vi "Open Text Log File.vi"(7 "Text Log File Type":refnum<class "Text Log File.lvclass">, 8 "error in (no error)":errorcluster, 9 "Disable Buffering (F)":bool, 10 "Operation":T1, 11 "File Path":path) -> (0 "error out":errorcluster, 3 "Text Log File out":refnum<class "Text Log File.lvclass">)   [LabVIEW 2015, in "Text Log File.lvclass"]
doc: "Opens a text file. Translate the file operation to the expected format and open the file. Set the file position to the end of the file in case we are appending to an existing file."
uses:
  Text Log File.lvclass
  Log File/Operation.ctl
  Log File/Log File Type.ctl
  Log File/Log File.lvclass/Log File.ctl
  Text Log File.lvclass/Text Log File.ctl
  Log File/Log File.lvclass
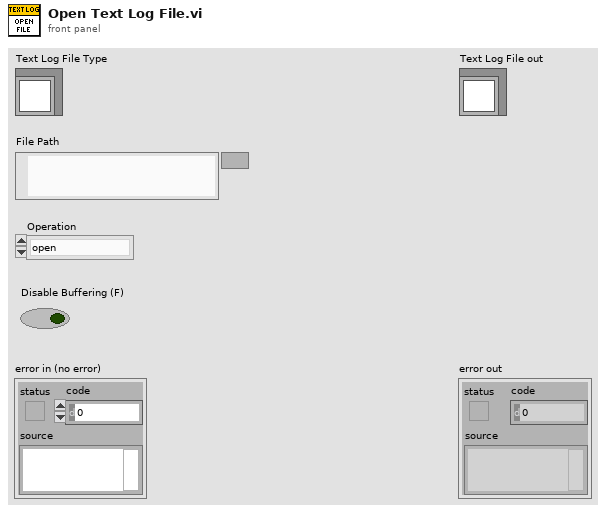
[diagram p1: front panel]
types:
  T1 = typedef "Log File.lvclass/Operation.ctl" = enum16{"open", "open or create", "create or replace", "create", "open (read-only)"}
  T2 = typedef "Log File.lvclass/Log File Type.ctl" = enum16{"Default", "TDMS", "Text"}
  T3 = enum16{"open", "replace", "create", "open or create", "replace or create", "replace or create with confirmation"}
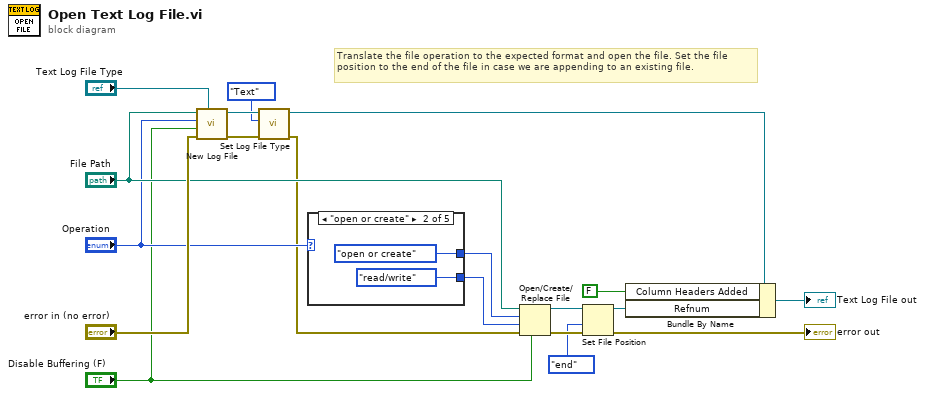
[diagram p0: block diagram]
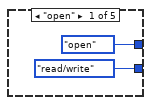
[diagram p2: hidden frame]
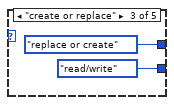
[diagram p3: hidden frame]
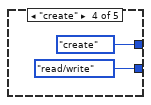
[diagram p4: hidden frame]
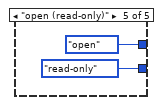
[diagram p5: hidden frame]
diagram:
  # "Translate the file operation to the expected format and open the file. Set the file position to the end of the file in case we are appending to an existing file."
  n1 = call "New Log File.vi"("Log File Type"="Text Log File Type", "error in (no error)"="error in (no error)", "Disable Buffering (F)"="Disable Buffering (F)", "Operation"="Operation", "File Path"="File Path") -> ("error out"=w4:errorcluster, "Log File out"=w5:refnum<class "Text Log File.lvclass">)  [unwired: 5 in]
  n2 = call "Set Log File Type.vi"("error in (no error)"=w4, "Log File Type"=Log_File_Type."Text", "Log File in"=w5) -> ("error out"=w3:errorcluster, "Log File out"=w2:refnum<class "Text Log File.lvclass">)  [unwired: 7 in]
  n3 = case shown="\"open or create\"" "Operation" {
    tunnel: [T3."open" ("operation (0:open)") T3."open or create" ("operation (0:open)") T3."replace or create" ("operation (0:open)") T3."create" ("operation (0:open)") T3."open" ("operation (0:open)")] -> w18
    tunnel: [enum16{"read/write", "read-only", "write-only"}."read/write" ("access (0:read/write)") enum16{"read/write", "read-only", "write-only"}."read/write" ("access (0:read/write)") enum16{"read/write", "read-only", "write-only"}."read/write" ("access (0:read/write)") enum16{"read/write", "read-only", "write-only"}."read/write" ("access (0:read/write)") enum16{"read/write", "read-only", "write-only"}."read-only" ("access (0:read/write)")] -> w17
    frame "open" {
    }
    frame "open or create" {
    }
    frame "create or replace" {
    }
    frame "create" {
    }
    frame "open (read-only)" {
    }
  }
  n4 = Open/Create/Replace File(file path (use dialog)="File Path", error in=w3, operation (0:open)=w18, access (0:read/write)=w17, disable buffering (F)="Disable Buffering (F)") -> (refnum out=w11:refnum<file>, error out=w10:errorcluster)  [unwired: 1 in, 1 out]
  n5 = Set File Position(refnum=w11, from (0:start)=enum16{"start", "end", "current"}."end", error in=w10) -> (refnum out=w8:refnum<file>, error out=→"error out":errorcluster)  [unwired: 1 in]
  n6 = Bundle By Name(cluster=w2, "Column Headers Added"=FALSE, "Refnum"=w8) -> (→"Text Log File out":refnum<class "Text Log File.lvclass">)
